vi "DO.vi"() -> ()   [LabVIEW 2021]
uses:
  <vilib>/FPGAPlugInAG/PCIe-7857/niLvFpga_Open_PCIe-7857.vi
  <vilib>/rvi/interface/common/dynamic/niFpgaDynamicAddResources.vi
  <vilib>/Utility/error.llb/Error Cluster From Error Code.vi
  <vilib>/rvi/errors/niLvFpgaAdjustHostInterfaceError.vi
  <vilib>/FPGAPlugInAG/Dynamic/niLvFpga_Run_Dynamic.vi
  <vilib>/FPGAPlugInAG/Dynamic/niLvFpga_Close_Dynamic.vi
  <vilib>/rvi/interface/nirviOpenFPGA/nirviOpenFPGA.xnode
  FPGA Bitfiles/lvfpga2_FPGATarget_FPGADigital_l3fEOdyPJeM.lvbitx
  <vilib>/rvi/interface/nirviMethod/nirviMethod.xnode
  <vilib>/rvi/interface/nirviReadWriteControl/nirviReadWriteControl.xnode
  <vilib>/rvi/interface/nirviCloseFPGA/nirviCloseFPGA.xnode
  NiFpgaLv.dll
  <vilib>/rvi/interface/Simulation/niFpgaSimulationCallBeginRW.vi
  <vilib>/FPGAPlugInAG/Dynamic/niLvFpga_WriteFifo_Dynamic.vi
  <vilib>/rvi/errors/niLvFpgaMergeErrorWithErrorCode.vi
panel:
  in  "Wait_time(uSec)":u32
  in  "Data":i16[](array[numeric])
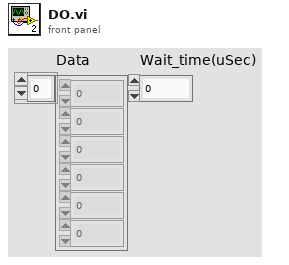
[diagram p1: front panel]
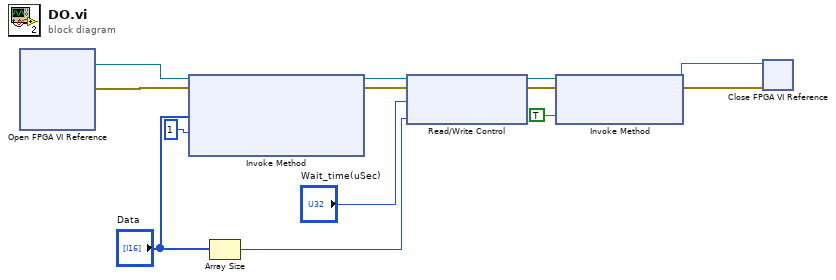
[diagram p0: block diagram]
diagram:
  n1 = xnode "Open FPGA VI Reference"() -> ("FPGA VI Reference Out"=w13:refnum<k20>, "error out"=w12:errorcluster)  [unwired: 2 in]
  n2 = xnode "Invoke Method"("FPGA VI Reference In"=w13, "error in"=w12, "Data"="Data", "Timeout (ms)"=1) -> ("FPGA VI Reference Out"=w10:refnum<k20>, "error out"=w7:errorcluster)  [unwired: 1 out]
  n3 = Array Size(array="Data") -> (size(s)=w1:i32)
  n4 = xnode "Read/Write Control"("FPGA VI Reference In"=w10, "error in"=w7, "Wait_time(uSec)"="Wait_time(uSec)", "Number_of_Steps"=w1) -> ("FPGA VI Reference Out"=w8:refnum<k20>, "error out"=w5:errorcluster)
  n5 = xnode "Invoke Method"("FPGA VI Reference In"=w8, "error in"=w5, "Wait Until Done (F)"=TRUE) -> ("FPGA VI Reference Out"=w6:refnum<k20>, "error out"=w3:errorcluster)
  n6 = xnode "Close FPGA VI Reference"("FPGA VI Reference In"=w6, "error in"=w3) -> ()  [unwired: 1 out]
